vi "Write New Card Ref.vi"(8 "error in (no error)":errorcluster, 10 "New Card":bool, 11 "WT1600 in":refnum<class "WT1600.lvclass">) -> (0 "error out":errorcluster, 3 "WT1600 out":refnum<class "WT1600.lvclass">)   [LabVIEW 2013, in "WT1600.lvlib" / "WT1600.lvclass"]
uses:
  WT1600.lvclass
  WT1600.lvclass/WT1600.ctl
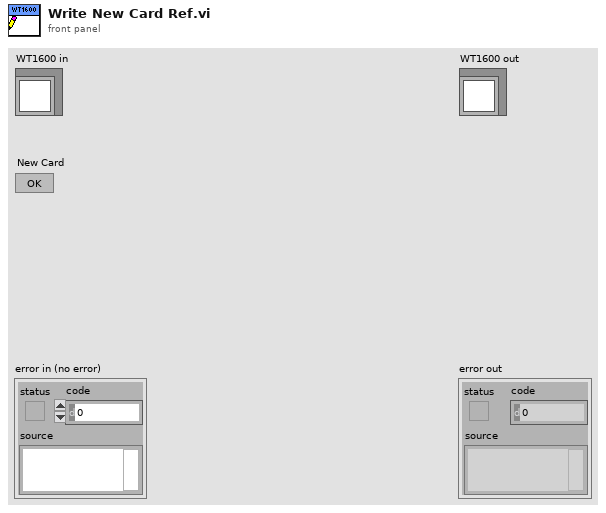
[diagram p1: front panel]
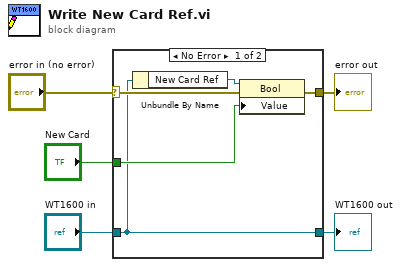
[diagram p0: block diagram]
diagram:
  n1 = case shown="No Error" "error in (no error)" {
    selector: "error in (no error)" -> [w9 w11]
    tunnel: [w8 w11] -> w4
    tunnel: [w6 w12] -> w2
    tunnel: "WT1600 in" -> [w6 w12]
    tunnel: "New Card" -> [w7 _]
    frame No Error {
      n2 = Unbundle By Name(w6) -> ("New Card Ref"=w10:refnum<vi>)
      n3 = property class="Bool"(reference=w10, error in=w9, "Value"=w7) -> (error out=w8:errorcluster)  [unwired: 1 out]
    }
    frame Error {
    }
  }
  "error out" <- w4
  "WT1600 out" <- w2
